vi "TargetGarbageCollect.vi"(5 "error in (no error)":errorcluster) -> (19 "error out":errorcluster)   [LabVIEW 2017, in "G#RemoteProxy.lvclass"]
doc: "Target performed a garbage collection. Kill all objects."
uses:
  G#RemoteProxy.lvclass
  C:/Program Files/National Instruments/LabVIEW 2017/vi.lib/addons/_AddQ/G#Object/G#Object.lvclass
  G#Object/G#Object.lvclass
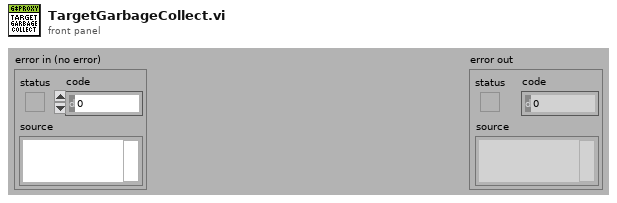
[diagram p1: front panel]
types:
  T1 = typedef "G#RemoteProxy.lvclass/ClassAttributesProxy.ctl" = cluster{"NoActiveProject":bool, "FullClassNames":string[], "FullClassPaths":path[], "RemoteRefs":refnum<class "G#Object.lvclass">[], "ProxyRefs":refnum<class "G#RemoteProxy.lvclass">[], "RemoteClassName":string[], "ProxyClassRefs":refnum<class "G#RemoteProxy.lvclass">[]}
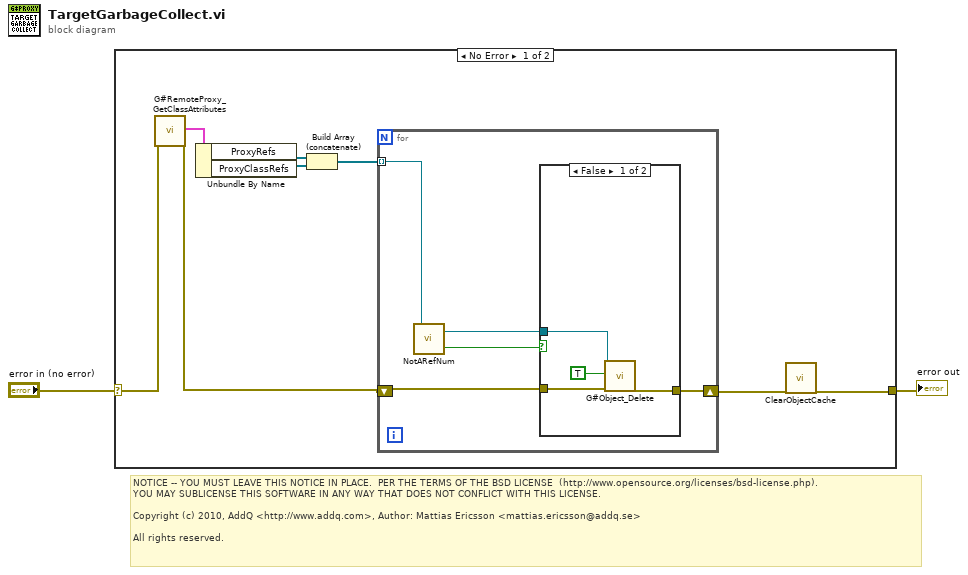
[diagram p0: block diagram]
diagram:
  # "NOTICE -- YOU MUST LEAVE THIS NOTICE IN PLACE.  PER THE TERMS OF THE BSD LICENSE  (http://www.opensource.org/licenses/bsd-license.php).\nYOU MAY SUBLICENSE THIS SOFTWARE IN ANY WAY THAT DOES NOT CONFLICT WITH THIS LICENSE.\n\nCopyright (c) 2010, AddQ <http://www.addq.com>, Author: Mattias Ericsson <mattias.ericsson@addq.se>\n\nAll rights reserved."
  n1 = case shown="No Error" "error in (no error)" {
    selector: "error in (no error)" -> [w10 w21]
    tunnel: [w3 w21] -> w1
    frame No Error {
      n2 = call "G#RemoteProxy_GetClassAttributes.vi"("error in (no error)"=w10) -> ("class attributes"=w9:T1, "error out"=w8:errorcluster)  [unwired: 15 in, 2 out]
      n3 = Unbundle By Name(w9) -> ("ProxyRefs"=w6:refnum<class "G#RemoteProxy.lvclass">[], "ProxyClassRefs"=w7:refnum<class "G#RemoteProxy.lvclass">[])
      n4 = Build Array (concatenate)(w6, w7) -> (w5:refnum<class "G#RemoteProxy.lvclass">[])
      n5 = for {
        shift-right: [w15] -> w4
        shift-left: w8 -> [w14]
        tunnel: w5 -> [w13] mode=indexing
        n6 = call-dynamic "NotARefNum.vi"("reference in"=w13) -> ("not a refnum?"=w11:bool, "reference out"=w12:refnum<class "G#RemoteProxy.lvclass">)  [unwired: 1 in]
        n7 = case shown="False" w11 {
          tunnel: [w19 w20] -> w15
          tunnel: w14 -> [w18 w20]
          tunnel: w12 -> [w17 _]
          frame False {
            n8 = call "G#Object_Delete.vi"("reference in"=w17, "force delete? (F)"=TRUE, "error in (no error)"=w18) -> ("error out"=w19:errorcluster)  [unwired: 15 in, 1 out]
          }
          frame True {
          }
        }
      }
      n9 = call "ClearObjectCache.vi"("error in (no error)"=w4) -> ("error out"=w3:errorcluster)  [unwired: 18 in]
    }
    frame Error {
    }
  }
  "error out" <- w1
